vi "Main.vi"() -> ()   [LabVIEW 2013]
uses:
  ctrl/TYPE User Event.ctl
  <vilib>/Utility/miscctls.llb/LVComboBoxStrsAndValuesArrayTypeDef.ctl
  <vilib>/Utility/error.llb/whitespace.ctl
  <vilib>/Utility/miscctls.llb/LVTextColorsTypeDef.ctl
  <vilib>/Utility/miscctls.llb/LVRowAndColumnUnsignedTypeDef.ctl
  <vilib>/Utility/file.llb/Read From Spreadsheet File (string).vi
panel:
  in  "Tab Control":enum32{"股票价格历史数据图", "股票实时数据图"}(tab)
  out "Date":string
  out "Name":string
  in  "Right":bool
  in  "Left":bool
  out "股票价格历史数据图":cluster{i32[], dbl[]}[](graph)
  in  "停止":bool
  out "时间":string
  out "当天股价实时曲线":dbl[][](graph)
  out "卖1竞价":dbl format="%.2g"
  out "买1竞价":dbl format="%.2g"
  out "卖1至5总量":dbl
  out "买1至5总量":dbl
  out "今日最低":dbl format="%.2f"
  out "今日最高":dbl format="%.2f"
  out "昨日收盘":dbl format="%.2f"
  out "今日开盘":dbl format="%.2f"
  out "当前股价":dbl format="%.2f"
  out "BuySellBar":cluster{dbl[], dbl[]}[](graph)
  out "当前%":dbl format="%.2g%%"
  in  "Up":bool
  in  "Down":bool
  in  "读取类型":enum32{"股票列表", "数据记录"}(tab)
  in  "股票代码查询":string(combo)
  in  "股票列表":i32(listbox)
  in  "股票文件列表":i32(listbox)
  out "股票数据路径":path
  in  "起始日期":timestamp=timestamp(3408258341.818551 s since 1904-01-01) format="%<%Y/%m/%d>T"
  in  "终止日期":timestamp format="%<%Y/%m/%d>T"
  # "起始日期"
  # "截止日期"
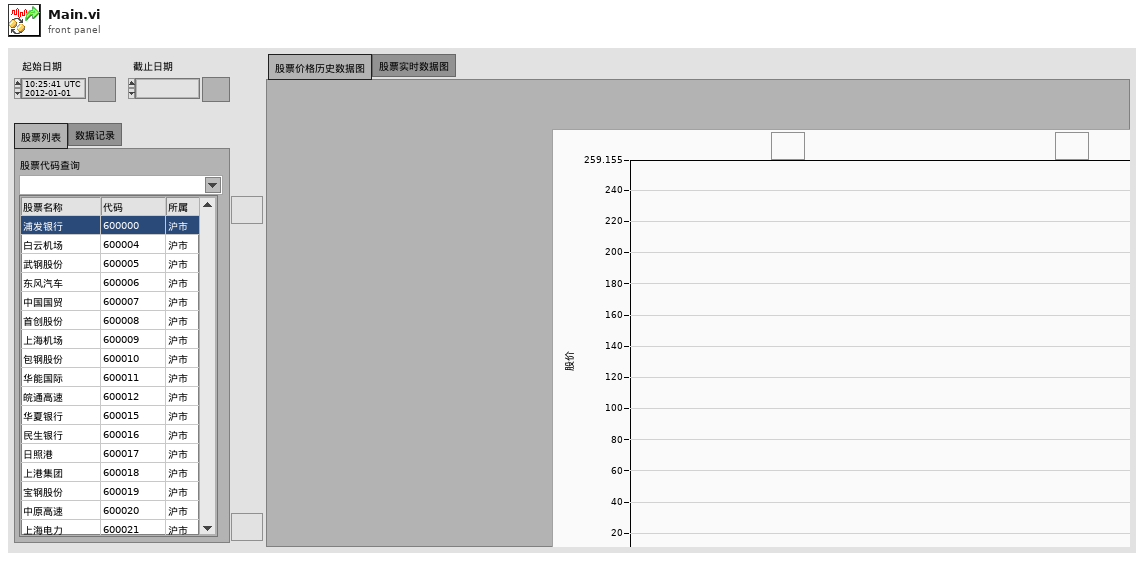
[diagram p1: front panel]
types:
  T1 = typedef "TYPE User Event.ctl" = cluster{"CMD":string, "Data":variant}
  T2 = cluster{"今日开盘":refnum<vi>, "昨日收盘":refnum<vi>, "当前股价":refnum<vi>, "今日最高":refnum<vi>, "今日最低":refnum<vi>, "买1竞价":refnum<vi>, "卖1竞价":refnum<vi>, "买1至5总量":refnum<vi>, "卖1至5总量":refnum<vi>, "当前%":refnum<vi>}
  T3 = typedef "LVComboBoxStrsAndValuesArrayTypeDef.ctl" = cluster{"String":string, "Value":string}[]
  T4 = typedef "LVTextColorsTypeDef.ctl" = cluster{"Text Color":u32, "Background Color":u32}
  T5 = typedef "LVRowAndColumnUnsignedTypeDef.ctl" = cluster{"Row":u32, "Column":u32}
  T6 = typedef "whitespace.ctl" = u16
  T7 = typedef "TYPE Price.ctl" = cluster{"Price":cluster{"Open":dbl, "Close":dbl, "Current":dbl, "High":dbl, "Low":dbl, "Buy1":dbl, "Sell1":dbl, "Total":dbl, "Account":dbl}, "Percent":dbl, "TotalBuy":dbl, "TotalSell":dbl, "TimeStamp":string}
  T8 = typedef "LVPoint32TypeDef.ctl" = cluster{"Horizontal":i32, "Vertical":i32}
  T9 = typedef "LVCursorListTypeDef.ctl" = cluster{"Name":string, "Color":u32, "Style":u8, "Point Style":u8, "Name Visible":bool, "Allow Drag":bool, "Cursor Mode":u32, "Plot":i32, "Index":i32, "Position":cluster{"X":dbl, "Y":dbl}, "X Scale":u32, "Y Scale":u32, "Watch Plots":i32[], "Watch All Plots":bool, "Plot Area":i32, "Label Offset":cluster{"X":dbl, "Y":dbl}}[]
  T10 = cluster{"Name":string, "Color":u32, "Style":u8, "Point Style":u8, "Name Visible":bool, "Allow Drag":bool, "Cursor Mode":u32, "Plot":i32, "Index":i32, "Position":cluster{"X":dbl, "Y":dbl}, "X Scale":u32, "Y Scale":u32, "Watch Plots":i32[], "Watch All Plots":bool, "Plot Area":i32, "Label Offset":cluster{"X":dbl, "Y":dbl}}
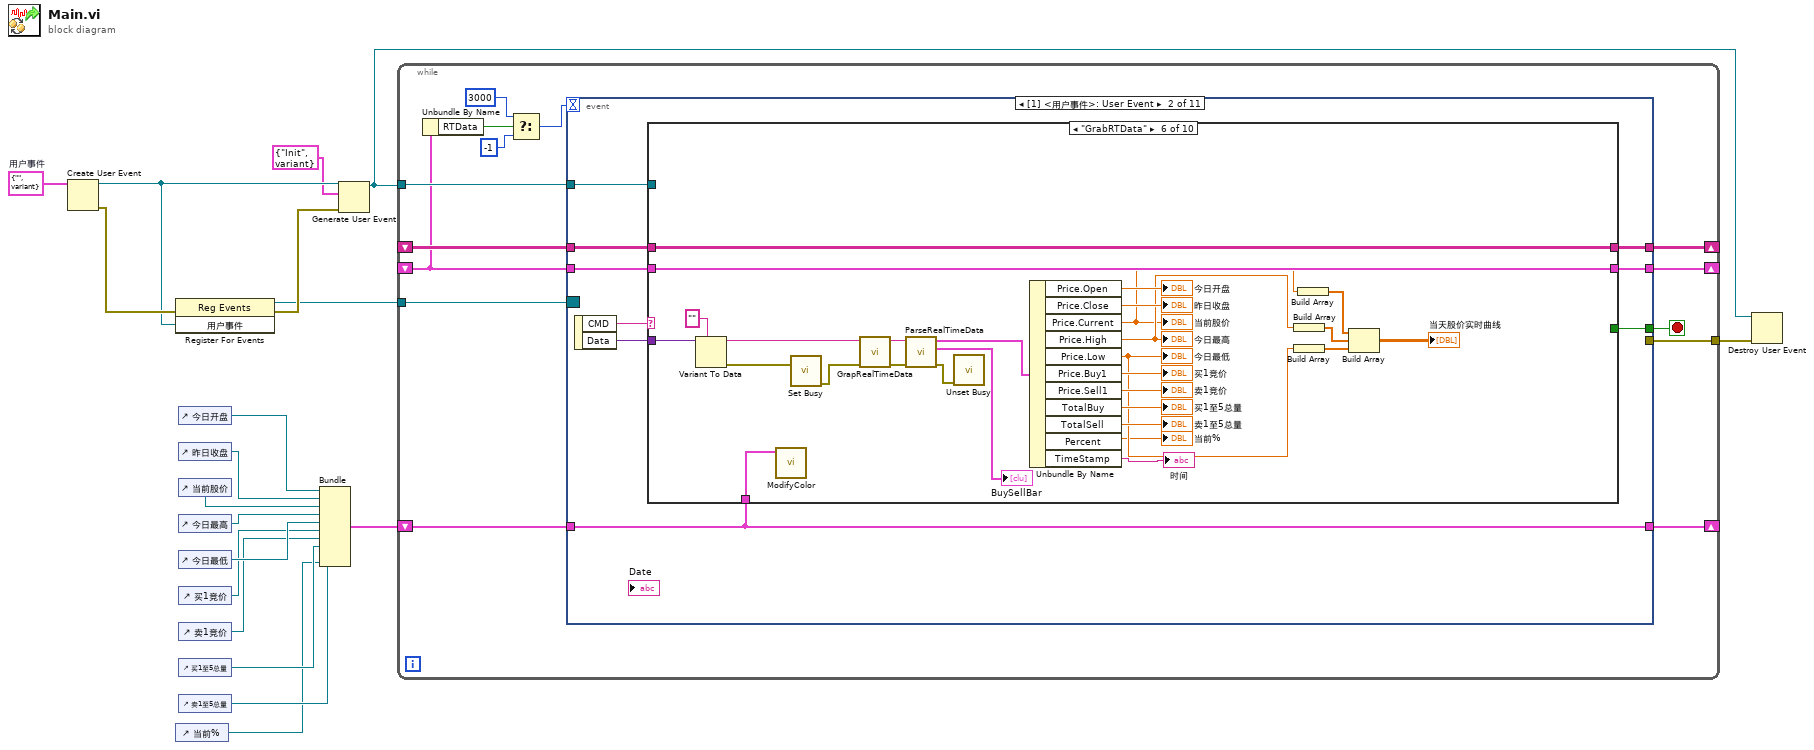
[diagram p0: block diagram]
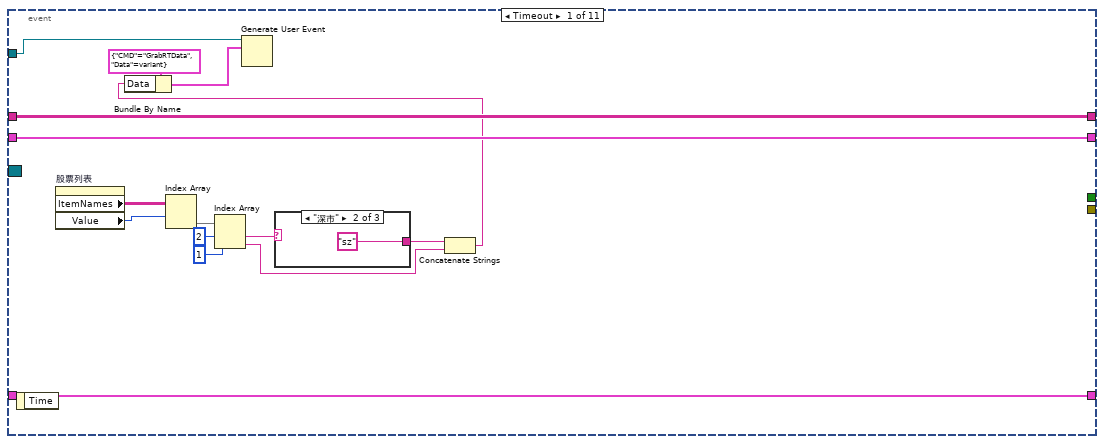
[diagram p2: hidden frame]
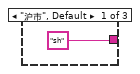
[diagram p3: hidden frame]
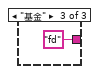
[diagram p4: hidden frame]
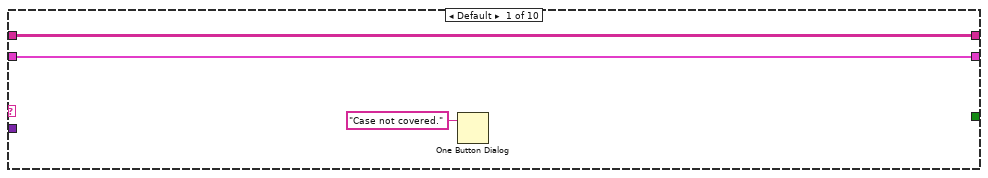
[diagram p5: hidden frame]
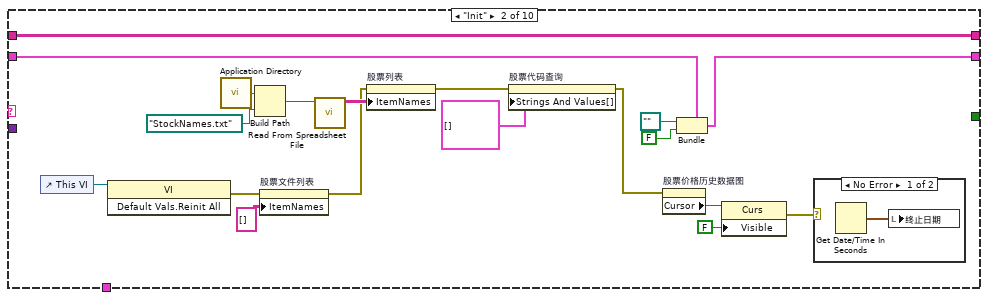
[diagram p6: hidden frame]
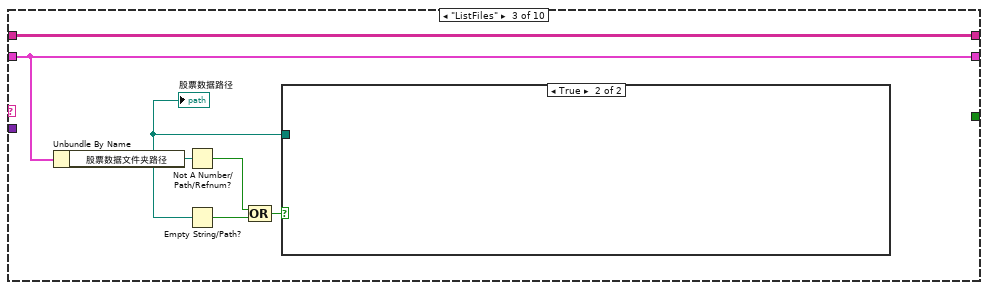
[diagram p8: hidden frame]
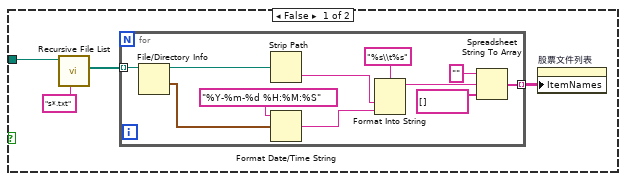
[diagram p9: hidden frame]
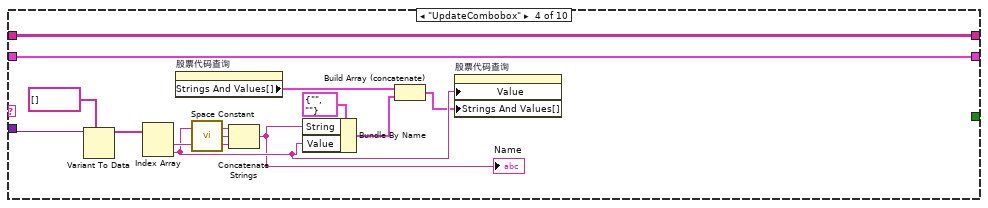
[diagram p10: hidden frame]
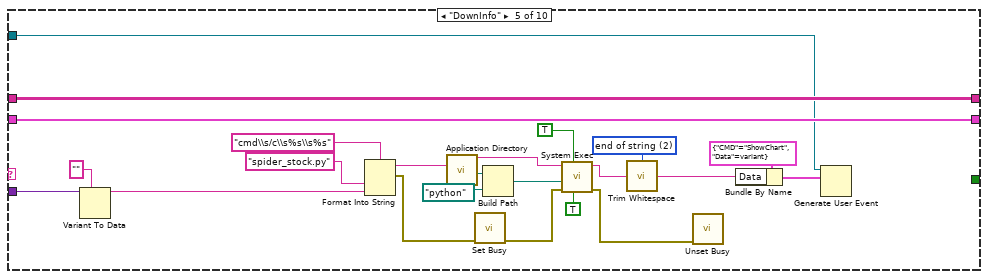
[diagram p11: hidden frame]
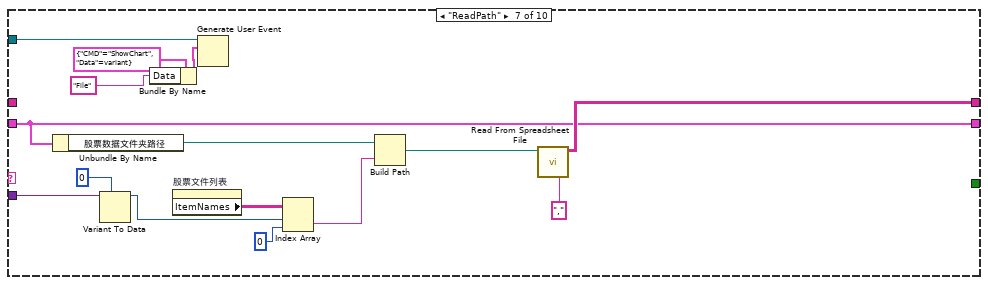
[diagram p12: hidden frame]
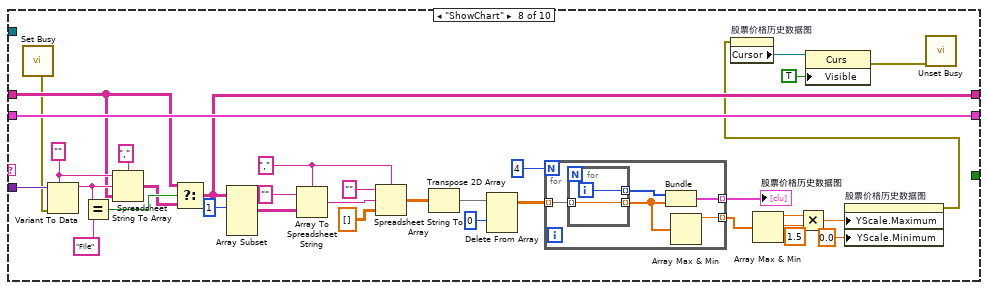
[diagram p13: hidden frame]
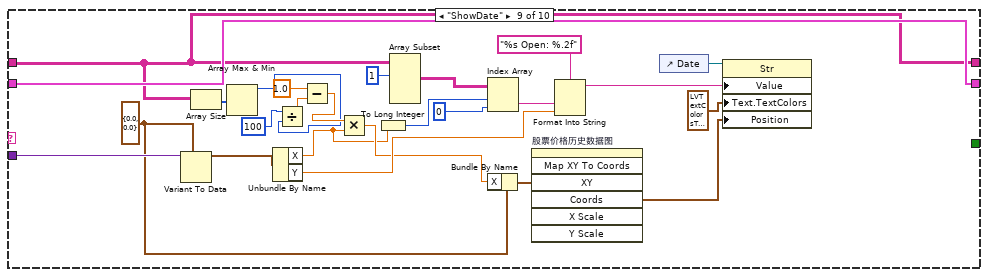
[diagram p14: hidden frame]
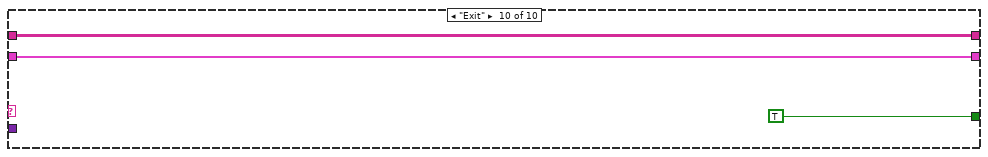
[diagram p15: hidden frame]
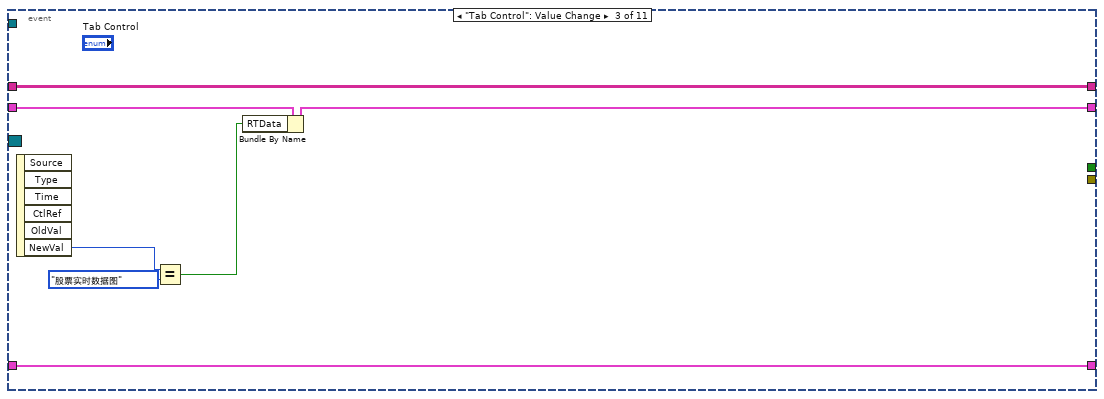
[diagram p16: hidden frame]
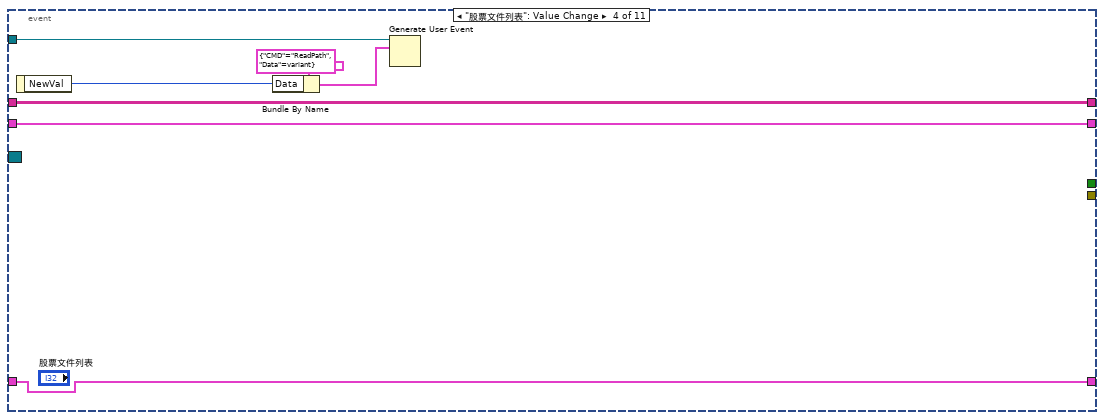
[diagram p17: hidden frame]
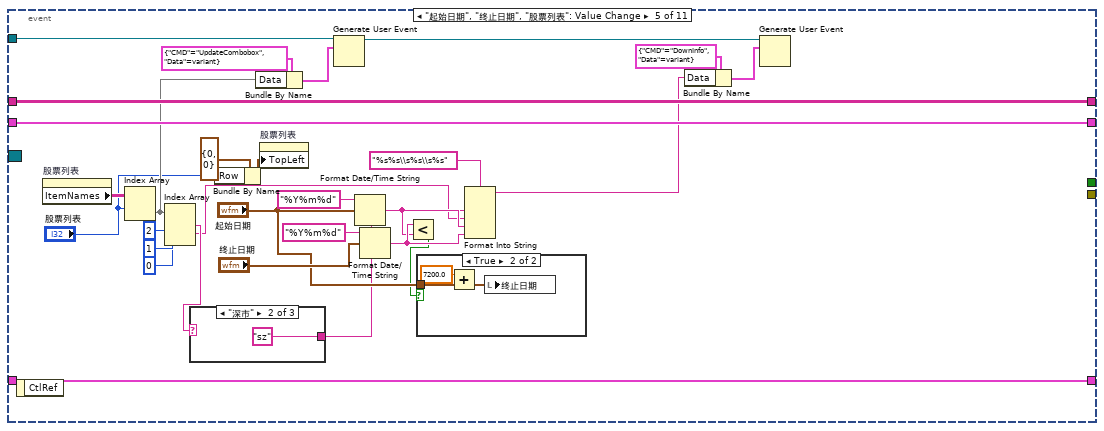
[diagram p18: hidden frame]
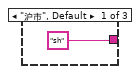
[diagram p19: hidden frame]
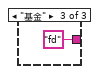
[diagram p20: hidden frame]
diagram:
  w15 = T1 {"CMD"="", "Data"=variant}  # 用户事件
  n1 = Create User Event(user event datatype=w15) -> (user event=w14:refnum<user-event>, error out=w18:errorcluster)  [unwired: 1 in]
  n2 = register-events(error in=w18, w14) -> (reference out=w17:refnum<event-registration>, error out=w19:errorcluster)  [unwired: 1 in]
  n3 = control-ref of="当前%"() -> (w1:refnum<vi>)
  n4 = control-ref of="今日开盘"() -> (w11:refnum<vi>)
  n5 = control-ref of="昨日收盘"() -> (w10:refnum<vi>)
  n6 = control-ref of="当前股价"() -> (w9:refnum<vi>)
  n7 = control-ref of="今日最高"() -> (w8:refnum<vi>)
  n8 = control-ref of="今日最低"() -> (w7:refnum<vi>)
  n9 = control-ref of="买1竞价"() -> (w6:refnum<vi>)
  n10 = control-ref of="卖1竞价"() -> (w5:refnum<vi>)
  n11 = control-ref of="买1至5总量"() -> (w4:refnum<vi>)
  n12 = control-ref of="卖1至5总量"() -> (w3:refnum<vi>)
  n13 = Bundle("今日开盘"=w11, "昨日收盘"=w10, "当前股价"=w9, "今日最高"=w8, "今日最低"=w7, "买1竞价"=w6, "卖1竞价"=w5, "买1至5总量"=w4, "卖1至5总量"=w3, "当前%"=w1) -> (w2:T2)  [unwired: 1 in]
  n14 = Generate User Event(user event=w14, event data cluster=T1 {"CMD"="Init", "Data"=variant} ("UsrEvent"), error in=w19) -> (user event out=w12:refnum<user-event>)  [unwired: 1 in, 1 out]
  n15 = while {
    shift-right: [w33] -> _
    shift-left: _ -> [w32]
    tunnel: w17 -> [w31]
    tunnel: w12 -> [w30]
    tunnel: [w29] -> w16
    shift-right: [w27] -> _
    shift-left: _ -> [w26]
    shift-right: [w21] -> _
    shift-left: w2 -> [w20]
    stop <- w28 stop-if-true
    n16 = Unbundle By Name(w26) -> ("RTData"=w24:bool)
    n17 = Select(t=3000, s=w24, f=-1) -> (s? t:f=w22:i32)
    n18 = event shown="[1] <用户事件>: User Event" {
      selector: w31 -> [_ _ _ _ _ _ _ _ _ _ _]
      dyn-events: _ -> [_ _ _ _ _ _ _ _ _ _ _]
      timeout: w22 -> [_ _ _ _ _ _ _ _ _ _ _]
      tunnel: [w48 w56 w257 w264 w293 w308 w324 w341 w358 w381 w390] -> w33
      tunnel: w32 -> [w48 w57 w257 w264 w293 w308 w324 w341 w358 w381 w390]
      tunnel: w30 -> [w44 w55 _ w262 w270 _ w313 w340 w354 _ w389]
      tunnel: [_ _ _ _ _ _ w312 _ _ _ _] -> w29
      tunnel: [_ w58 _ _ _ _ _ _ _ _ _] -> w28
      tunnel: w26 -> [w47 w54 w256 w259 w292 w307 w320 w336 w357 w380 w387]
      tunnel: [w47 w53 w253 w259 w292 w307 w321 w336 w357 w380 w387] -> w27
      tunnel: [w34 w52 w251 w258 w265 w300 w310 w334 w342 w375 w386] -> w21
      tunnel: w20 -> [w34 w52 w251 w258 w265 w300 w310 w334 w342 w375 w386]
      event Timeout {
        n19 = event-data() -> ()  [unwired: 1 in, 1 out]
        n20 = property on="股票列表" class="MCListbox (strict)"() -> ("ItemNames"=w43:string[][], "Value"=w42:i32)  [unwired: 2 in, 2 out]
        n21 = Index Array(array=w43, index (row)=w42) -> (element=w41:string[])  [unwired: 1 in]
        n22 = Index Array(array=w41, index #1=2 ("index"), index #2=1 ("index")) -> (element #1=w39:string, element #2=w36:string)
        n23 = case shown="\"深市\"" w39 {
          tunnel: ["sh" ("代码") "sz" ("代码") "fd" ("代码")] -> w37
          frame "沪市", Default {
          }
          frame "深市" {
          }
          frame "基金" {
          }
        }
        n24 = Concatenate Strings(w37, w36) -> (w35:string)
        n25 = Bundle By Name(cluster=T1 {"CMD"="GrabRTData", "Data"=variant} ("UsrEvent"), "Data"=w35) -> (w45:T1)
        n26 = Generate User Event(user event=w44, event data cluster=w45) -> ()  [unwired: 2 in, 2 out]
      }
      event User Event {
        n27 = event-data() -> ("CMD"=w60:string, "Data"=w59:variant)  [unwired: 1 in]
        n28 = case shown="\"GrabRTData\"" w60 {
          tunnel: w57 -> [w63 w82 w89 w117 w139 w167 _ w194 w231 w249]
          tunnel: w59 -> [_ _ _ w115 w133 w164 w180 w200 w246 _]
          tunnel: [_ _ _ _ _ _ _ _ _ TRUE] -> w58
          tunnel: [w63 w82 w89 w117 w139 w167 w182 w192 w231 w249] -> w56
          tunnel: w55 -> [_ _ _ _ w129 _ w181 _ _ _]
          tunnel: w54 -> [w62 w78 w88 w116 w138 w166 w174 w203 w240 w248]
          tunnel: [w62 w77 w88 w116 w138 w166 w174 w203 w240 w248] -> w53
          tunnel: w52 -> [_ _ _ _ _ w142 _ _ _ _]
          frame Default {
            n29 = One Button Dialog(message="Case not covered.") -> ()  [unwired: 1 in, 1 out]
          }
          frame "Init" {
            n30 = control-ref of="This VI"() -> (w80:refnum<vi>)
            n31 = invoke class="VI" method="Default Vals.Reinit All"(reference=w80) -> (error out=w79:errorcluster)  [unwired: 2 in, 2 out]
            n32 = call <vilib>:"Application Directory.vi"() -> ("Application Directory"=w71:path)
            n33 = Build Path(base path=w71, name or relative path=path "StockNames.txt" ("file path (dialog if empty)")) -> (appended path=w69:path)
            n34 = property on="股票文件列表" class="MCListbox (strict)"(error in=w79, "ItemNames"=string[][] [] ("Item Names")) -> (error out=w66:errorcluster)  [unwired: 1 in, 1 out]
            n35 = call-poly <vilib>:"Read From Spreadsheet File.vi"("file path (dialog if empty)"=w69) -> ("all rows"=w72:string[][])  [unwired: 6 in, 4 out]
            n36 = property on="股票列表" class="MCListbox (strict)"(error in=w66, "ItemNames"=w72) -> (error out=w67:errorcluster)  [unwired: 1 in, 1 out]
            n37 = property on="股票代码查询" class="CmbBox"(error in=w67, "Strings And Values[]"=T3 [] ("Strings And Values []")) -> (error out=w65:errorcluster)  [unwired: 1 in, 1 out]
            n38 = property on="股票价格历史数据图" class="XYGraph (strict)"(error in=w65) -> ("Cursor"=w75:refnum<vi>)  [unwired: 1 in, 2 out]
            n39 = Bundle(cluster=w78, "股票数据文件夹路径"=path "", "RTData"=FALSE) -> (w77:cluster{"股票数据文件夹路径":path, "RTData":bool})
            n40 = property class="Curs"(reference=w75, "Visible"=FALSE) -> (error out=w73:errorcluster)  [unwired: 1 in, 1 out]
            n41 = case shown="No Error" w73 {
              frame No Error {
                n42 = Get Date/Time In Seconds() -> (seconds since 1Jan1904=w83:timestamp)
                n43 = local write "终止日期"(w83) -> ()
              }
              frame Error {
              }
            }
          }
          frame "ListFiles" {
            n44 = Unbundle By Name(w88) -> ("股票数据文件夹路径"=w84:path)
            "股票数据路径" <- w84
            n45 = Not A Number/Path/Refnum?(number/path/refnum=w84) -> (NaN/Path/Refnum?=w86:bool)
            n46 = Empty String/Path?(string/path=w84) -> (empty?=w87:bool)
            n47 = Compound Arithmetic op=OR(w86, w87) -> (w85:bool)
            n48 = case shown="True" w85 {
              tunnel: w84 -> [w90 _]
              frame False {
                n49 = call <vilib>:"Recursive File List.vi"("pattern"="s*.txt", "Folder Path"=w90) -> ("All Files in Dir"=w92:path[])  [unwired: 5 in, 4 out]
                n50 = for {
                  tunnel: w92 -> [w104] mode=indexing
                  tunnel: [w98] -> w91 mode=indexing
                  n51 = File/Directory Info(path=w104) -> (path out=w103:path, last mod=w102:timestamp)  [unwired: 1 in, 5 out]
                  n52 = Strip Path(path=w103) -> (name=w96:string)  [unwired: 1 out]
                  n53 = Format Date/Time String(time format string (%c)="%Y-%m-%d %H:%M:%S", seconds (now)=w102) -> (date/time string=w95:string)  [unwired: 1 in]
                  n54 = Format Into String(format string="%s\\t%s", w96, w95) -> (resulting string=w99:string)  [unwired: 2 in, 1 out]
                  n55 = Spreadsheet String To Array(format string="", spreadsheet string=w99, array type (2D Dbl)=string[] []) -> (array=w98:string[])  [unwired: 1 in]
                }
                n56 = property on="股票文件列表" class="MCListbox (strict)"("ItemNames"=w91) -> ()  [unwired: 2 in, 2 out]
              }
              frame True {
              }
            }
          }
          frame "UpdateCombobox" {
            n57 = Variant To Data(type=string[] [] ("subarray"), Variant=w115) -> (data=w113:string[])  [unwired: 1 in, 1 out]
            n58 = Index Array(array=w113) -> (element #1=w109:string, element #2=w107:string)  [unwired: 2 in]
            n59 = property on="股票代码查询" class="CmbBox"() -> ("Strings And Values[]"=w111:T3)  [unwired: 2 in, 2 out]
            n60 = call <vilib>:"Space Constant.vi"() -> ("String"=w108:string)
            n61 = Concatenate Strings(w107, w108, w109) -> (w105:string)
            "Name" <- w105
            n62 = Bundle By Name(cluster=cluster{"String":string, "Value":string} {"String"="", "Value"=""}, "String"=w105, "Value"=w107) -> (w110:cluster{"String":string, "Value":string})
            n63 = Build Array (concatenate)(w111, w110) -> (w106:T3)
            n64 = property on="股票代码查询" class="CmbBox"("Value"=w107, "Strings And Values[]"=w106) -> ()  [unwired: 2 in, 2 out]
          }
          frame "DownInfo" {
            w124 = T6 2 items=["both", "start of string", "end of string"] ("location (both)")
            n65 = Variant To Data(type="", Variant=w133) -> (data=w131:string)  [unwired: 1 in, 1 out]
            n66 = Format Into String(format string="cmd\\s/c\\s%s\\s%s", "spider_stock.py" ("input 1"), w131) -> (resulting string=w134:string, error out=w123:errorcluster)  [unwired: 2 in]
            n67 = call <vilib>:"Application Directory.vi"() -> ("Application Directory"=w120:path)
            n68 = call <vilib>:"Set Busy.vi"("error in (no error)"=w123) -> ("error out"=w122:errorcluster)  [unwired: 9 in, 1 out]
            n69 = Build Path(base path=w120, name or relative path=path "python" ("working directory")) -> (appended path=w118:path)
            n70 = call <vilib>:"System Exec.vi"("run minimized? (F)"=TRUE, "wait until completion? (T)"=TRUE, "error in (no error)"=w122, "working directory"=w118, "command line"=w134) -> ("error out"=w121:errorcluster, "standard output"=w126:string)  [unwired: 3 in, 2 out]
            n71 = call <vilib>:"Trim Whitespace.vi"("string"=w126, "location (both)"=w124) -> ("trimmed string"=w125:string)
            n72 = call <vilib>:"Unset Busy.vi"("error in (no error)"=w121) -> ()  [unwired: 10 in, 1 out]
            n73 = Bundle By Name(cluster=T1 {"CMD"="ShowChart", "Data"=variant} ("UsrEvent"), "Data"=w125) -> (w128:T1)
            n74 = Generate User Event(user event=w129, event data cluster=w128) -> ()  [unwired: 2 in, 2 out]
          }
          frame "GrabRTData" {
            n75 = Variant To Data(type="", Variant=w164) -> (data=w163:string, error out=w146:errorcluster)  [unwired: 1 in]
            n76 = call "ModifyColor.vi"("ControlRefsIn"=w142) -> ()  [unwired: 10 in, 1 out]
            n77 = call <vilib>:"Set Busy.vi"("error in (no error)"=w146) -> ("error out"=w145:errorcluster)  [unwired: 9 in, 1 out]
            n78 = call "GrapRealTimeData.vi"("error in (no error)"=w145, "Code"=w163) -> ("error out"=w144:errorcluster, "Grab Data"=w162:string)  [unwired: 8 in]
            n79 = call "ParseRealTimeData.vi"("error in (no error)"=w144, "Raw Data"=w162) -> ("error out"=w143:errorcluster, "BuySellBar"=→"BuySellBar":cluster{dbl[], dbl[]}[], "Price"=w161:T7)  [unwired: 7 in]
            n80 = call <vilib>:"Unset Busy.vi"("error in (no error)"=w143) -> ()  [unwired: 10 in, 1 out]
            n81 = Unbundle By Name(w161) -> ("Price.Open"=→"今日开盘":dbl, "Price.Close"=→"昨日收盘":dbl, "Price.Current"=w149:dbl, "Price.High"=w154:dbl, "Price.Low"=w153:dbl, "Price.Buy1"=→"买1竞价":dbl, "Price.Sell1"=→"卖1竞价":dbl, "TotalBuy"=→"买1至5总量":dbl, "TotalSell"=→"卖1至5总量":dbl, "Percent"=→"当前%":dbl, "TimeStamp"=→"时间":string)
            "当前股价" <- w149
            "今日最低" <- w153
            "今日最高" <- w154
            n82 = Build Array(w154) -> (w151:dbl[])
            n83 = Build Array(w153) -> (w152:dbl[])
            n84 = Build Array(w149) -> (w148:dbl[])
            n85 = Build Array(w148, w151, w152) -> (→"当天股价实时曲线":dbl[][])
          }
          frame "ReadPath" {
            n86 = Unbundle By Name(w174) -> ("股票数据文件夹路径"=w173:path)
            n87 = Variant To Data(type=0, Variant=w180) -> (data=w177:i32)  [unwired: 1 in, 1 out]
            n88 = Bundle By Name(cluster=T1 {"CMD"="ShowChart", "Data"=variant} ("UsrEvent"), "Data"="File" ("CMD")) -> (w169:T1)
            n89 = property on="股票文件列表" class="MCListbox (strict)"() -> ("ItemNames"=w178:string[][])  [unwired: 2 in, 2 out]
            n90 = Generate User Event(user event=w181, event data cluster=w169) -> ()  [unwired: 2 in, 2 out]
            n91 = Index Array(array=w178, index (row)=w177, index (col)=0 ("disabled index (col)")) -> (element=w175:string)
            n92 = Build Path(base path=w173, name or relative path=w175) -> (appended path=w172:path)
            n93 = call-poly <vilib>:"Read From Spreadsheet File.vi"("delimiter (\\t)"="," ("delimiter (\\t)"), "file path (dialog if empty)"=w172) -> ("all rows"=w182:string[][])  [unwired: 5 in, 4 out]
          }
          frame "ShowChart" {
            w199 = "" ("Date")
            w206 = "," ("delimiter (Tab)")
            n94 = call <vilib>:"Set Busy.vi"() -> ("error out"=w184:errorcluster)  [unwired: 10 in, 1 out]
            n95 = Variant To Data(error in=w184, type=w199, Variant=w200) -> (data=w197:string)  [unwired: 1 out]
            n96 = Equal?(x=w197, y="File") -> (x = y?=w195:bool)
            n97 = Spreadsheet String To Array(delimiter (Tab)=",", format string=w199, spreadsheet string=w197, array type (2D Dbl)=w194) -> (array=w193:string[][])
            n98 = Select(t=w194, s=w195, f=w193) -> (s? t:f=w192:string[][])
            n99 = Array Subset(array=w192, index (row)=1 ("index")) -> (w215:string[][])  [unwired: 3 in]
            n100 = Array To Spreadsheet String(delimiter (Tab)=w206, array=w215, 3:"" ("format string")) -> (spreadsheet string=w205:string)
            n101 = Spreadsheet String To Array(delimiter (Tab)=w206, format string="", spreadsheet string=w205, array type (2D Dbl)=dbl[][] []) -> (array=w210:dbl[][])
            n102 = Transpose 2D Array(2D array=w210) -> (transposed array=w213:dbl[][])
            n103 = Delete From Array(array=w213, index (row)=0) -> (array with subset deleted=w190:dbl[][])  [unwired: 2 in, 1 out]
            n104 = for {
              N: 4 -> [_]
              tunnel: w190 -> [w220] mode=indexing
              tunnel: [w218] -> w211 mode=indexing
              tunnel: [w216] -> w189 mode=indexing
              n105 = for {
                tunnel: w220 -> [w221] mode=indexing
                tunnel: [w221] -> w217 mode=indexing
                tunnel: [w222] -> w219 mode=indexing
                i -> [w222]
              }
              n106 = Bundle(w219, w217) -> (w218:cluster{i32[], dbl[]})  [unwired: 1 in]
              n107 = Array Max & Min(array=w217) -> (max value=w216:dbl)  [unwired: 3 out]
            }
            "股票价格历史数据图" <- w211
            n108 = Array Max & Min(array=w189) -> (max value=w188:dbl)  [unwired: 3 out]
            n109 = Multiply(x=w188, y=1.5) -> (x*y=w187:dbl)
            n110 = property on="股票价格历史数据图" class="XYGraph (strict)"("YScale.Maximum"=w187, "YScale.Minimum"=0.0 ("Y Scale.Range:Minimum")) -> (error out=w185:errorcluster)  [unwired: 2 in, 1 out]
            n111 = property on="股票价格历史数据图" class="XYGraph (strict)"(error in=w185) -> ("Cursor"=w202:refnum<vi>)  [unwired: 1 in, 2 out]
            n112 = property class="Curs"(reference=w202, "Visible"=TRUE) -> (error out=w183:errorcluster)  [unwired: 1 in, 1 out]
            n113 = call <vilib>:"Unset Busy.vi"("error in (no error)"=w183) -> ()  [unwired: 10 in, 1 out]
          }
          frame "ShowDate" {
            w234 = cluster{"X":dbl, "Y":dbl} {"X"=0.0, "Y"=0.0} ("CursLoc")
            n114 = Variant To Data(type=w234, Variant=w246) -> (data=w233:cluster{"X":dbl, "Y":dbl})  [unwired: 1 in, 1 out]
            n115 = Array Size(array=w231) -> (size(s)=w230:i32[])
            n116 = Array Max & Min(array=w230) -> (max value=w223:i32)  [unwired: 3 out]
            n117 = Unbundle By Name(w233) -> ("X"=w225:dbl, "Y"=w232:dbl)
            n118 = Divide(x=100, y=w223) -> (x/y=w228:dbl)
            n119 = Subtract(x=1.0, y=w228) -> (x-y=w227:dbl)
            n120 = Multiply(x=w227, y=w225) -> (x*y=w226:dbl)
            n121 = To Long Integer(number=w225) -> (32bit integer=w242:i32)
            n122 = Array Subset(array=w231, index (row)=1 ("index")) -> (w243:string[][])  [unwired: 3 in]
            n123 = Index Array(array=w243, index (row)=w242, index (col)=0 ("disabled index (col)")) -> (element=w237:string)
            n124 = Bundle By Name(cluster=w234, "X"=w226) -> (w235:cluster{"X":dbl, "Y":dbl})
            n125 = invoke on="股票价格历史数据图" class="XYGraph (strict)" method="Map XY To Coords"("XY"=w235) -> ("Coords"=w239:T8)  [unwired: 6 in, 6 out]
            n126 = Format Into String(format string="%s Open: %.2f", w237, w232) -> (resulting string=w238:string)  [unwired: 2 in, 1 out]
            n127 = control-ref of="Date"() -> (w247:refnum<vi>)
            n128 = property class="Str"(reference=w247, "Value"=w238, "Text.TextColors"=T4 {"Text Color"=16777222, "Background Color"=16777216} ("Text.Text Colors"), "Position"=w239) -> ()  [unwired: 1 in, 2 out]
          }
          frame "Exit" {
          }
        }
      }
      event "Tab Control": Value Change {
        n129 = event-data() -> ("NewVal"=w255:enum32{"股票价格历史数据图", "股票实时数据图"})  [unwired: 1 in, 5 out]
        n130 = Equal?(x=w255, y=enum32{"股票价格历史数据图", "股票实时数据图"}."股票实时数据图") -> (x = y?=w252:bool)
        n131 = Bundle By Name(cluster=w256, "RTData"=w252) -> (w253:cluster{"股票数据文件夹路径":path, "RTData":bool})
      }
      event "股票文件列表": Value Change {
        n132 = event-data() -> ("NewVal"=w260:i32)  [unwired: 1 in]
        n133 = Bundle By Name(cluster=T1 {"CMD"="ReadPath", "Data"=variant} ("UsrEvent"), "Data"=w260) -> (w261:T1)
        n134 = Generate User Event(user event=w262, event data cluster=w261) -> ()  [unwired: 2 in, 2 out]
      }
      event "起始日期", "终止日期", "股票列表": Value Change {
        n135 = event-data() -> ()  [unwired: 1 in, 1 out]
        n136 = property on="股票列表" class="MCListbox (strict)"() -> ("ItemNames"=w280:string[][])  [unwired: 2 in, 2 out]
        n137 = Index Array(array=w280, index (row)="股票列表") -> (element=w271:string[])  [unwired: 1 in]
        n138 = Index Array(array=w271, index #1=2 ("index"), index #2=1 ("index"), index #3=0 ("index")) -> (element #1=w277:string, element #2=w274:string)  [unwired: 1 out]
        n139 = case shown="\"深市\"" w277 {
          tunnel: ["sh" ("代码") "sz" ("代码") "fd" ("代码")] -> w276
          frame "沪市", Default {
          }
          frame "深市" {
          }
          frame "基金" {
          }
        }
        n140 = Bundle By Name(cluster=T5 {"Row"=0, "Column"=0} ("Top Left Visible Cell"), "Row"="股票列表") -> (w267:T5)
        n141 = Bundle By Name(cluster=T1 {"CMD"="UpdateCombobox", "Data"=variant} ("UsrEvent"), "Data"=w271) -> (w272:T1)
        n142 = property on="股票列表" class="MCListbox (strict)"("TopLeft"=w267) -> ()  [unwired: 2 in, 2 out]
        n143 = Generate User Event(user event=w270, event data cluster=w272) -> (user event out=w269:refnum<user-event>)  [unwired: 2 in, 1 out]
        n144 = Format Date/Time String(time format string (%c)="%Y%m%d", seconds (now)="起始日期") -> (date/time string=w281:string)  [unwired: 1 in]
        n145 = Format Date/Time String(time format string (%c)="%Y%m%d", seconds (now)="终止日期") -> (date/time string=w284:string)  [unwired: 1 in]
        n146 = Less?(x=w284, y=w281) -> (x < y?=w282:bool)
        n147 = case shown="True" w282 {
          tunnel: "起始日期" -> [_ w299]
          frame False {
          }
          frame True {
            n148 = Add(x=7200.0, y=w299) -> (x+y=w298:timestamp)
            n149 = local write "终止日期"(w298) -> ()
          }
        }
        n150 = Format Into String(format string="%s%s\\s%s\\s%s", w276, w274, w281, w284) -> (resulting string=w285:string)  [unwired: 2 in, 1 out]
        n151 = Bundle By Name(cluster=T1 {"CMD"="DownInfo", "Data"=variant} ("UsrEvent"), "Data"=w285) -> (w286:T1)
        n152 = Generate User Event(user event=w269, event data cluster=w286) -> ()  [unwired: 2 in, 2 out]
      }
      event "股票代码查询": Value Change {
        n153 = event-data() -> ()  [unwired: 1 in, 1 out]
        n154 = property on="股票列表" class="MCListbox (strict)"() -> ("ItemNames"=w302:string[][])  [unwired: 2 in, 2 out]
        n155 = Index Array(array=w302, index (col)=1 ("disabled index (col)")) -> (element=w303:string[])  [unwired: 1 in]
        n156 = Search 1D Array(1D array=w303, element="股票代码查询") -> (index of element=w301:i32)  [unwired: 1 in]
        n157 = Greater Or Equal To 0?(x=w301) -> (x >= 0?=w304:bool)
        n158 = case shown="True" w304 {
          tunnel: w301 -> [_ w309]
          frame False {
          }
          frame True {
            n159 = property on="股票列表" class="MCListbox (strict)"("Val(Sgnl)"=w309) -> ()  [unwired: 2 in, 2 out]
          }
        }
      }
      event "读取类型": Value Change {
        n160 = event-data() -> ("NewVal"=w323:enum32{"股票列表", "数据记录"})  [unwired: 1 in]
        n161 = Unbundle By Name(w320) -> ("股票数据文件夹路径"=w317:path)
        n162 = Not A Number/Path/Refnum?(number/path/refnum=w317) -> (NaN/Path/Refnum?=w318:bool)
        n163 = Empty String/Path?(string/path=w317) -> (empty?=w319:bool)
        n164 = Compound Arithmetic op=OR(w318, w319) -> (w316:bool)
        n165 = Equal?(x=enum32{"股票列表", "数据记录"}."数据记录", y=w323) -> (x = y?=w314:bool)
        n166 = Compound Arithmetic op=AND(w316, w314) -> (w315:bool)
        n167 = case shown="True" w315 {
          tunnel: w320 -> [w329 w332]
          tunnel: [w329 w331] -> w321
          tunnel: [_ w330] -> w311
          frame False {
          }
          frame True {
            n168 = call "File Dialog"() -> ("selected path"=w333:path, "error out"=w330:errorcluster)  [unwired: 12 in, 2 out]
            n169 = Bundle By Name(cluster=w332, "股票数据文件夹路径"=w333) -> (w331:cluster{"股票数据文件夹路径":path, "RTData":bool})
          }
        }
        n170 = case shown="True" w314 {
          tunnel: w313 -> [_ w328]
          tunnel: [_ w327] -> w312
          tunnel: w311 -> [_ w325]
          frame False {
          }
          frame True {
            n171 = Generate User Event(user event=w328, event data cluster=T1 {"CMD"="ListFiles", "Data"=variant} ("UsrEvent"), error in=w325) -> (error out=w327:errorcluster)  [unwired: 1 in, 1 out]
          }
        }
      }
      event "股票价格历史数据图": Cursor Move {
        n172 = event-data() -> ("CursLoc"=w335:cluster{"X":dbl, "Y":dbl})  [unwired: 1 in]
        n173 = Bundle By Name(cluster=T1 {"CMD"="", "Data"=variant} ("UsrEvent"), "CMD"="ShowDate", "Data"=w335) -> (w337:T1)
        n174 = Generate User Event(user event=w340, event data cluster=w337) -> ()  [unwired: 2 in, 2 out]
      }
      event "Left", "Right": Value Change {
        n175 = event-data() -> ("CtlRef"=w353:refnum<vi>)  [unwired: 1 in, 3 out]
        n176 = property class="Bool"(reference=w353) -> ("Label.Text"=w352:string)  [unwired: 1 in, 2 out]
        n177 = property on="股票价格历史数据图" class="XYGraph (strict)"() -> (error out=w351:errorcluster, "CrsrList"=w348:T9)  [unwired: 2 in, 1 out]
        n178 = for {
          tunnel: w352 -> [w365]
          tunnel: [w364] -> w347 mode=indexing
          tunnel: w348 -> [w361] mode=indexing
          shift-right: [w362] -> w350
          shift-left: w351 -> [w363]
          tunnel: [w360] -> w346
          tunnel: [w359] -> w343
          n179 = in-place {
            in-place-border: w365 -> [w370]
            in-place-border: w363 -> [w368]
            in-place-border: [w368] -> w362
            in-place-border: [w367] -> w360
            in-place-border: [w366] -> w359
            n180 = in-place-cluster #1(w361) -> ("Position.X"=w369:dbl, "Position.Y"=w366:dbl)
            n181 = case shown="\"Right\", Default" w370 {
              tunnel: w369 -> [w372 w374]
              tunnel: [w371 w373] -> w367
              frame "Right", Default {
                n182 = Increment(x=w372) -> (x+1=w371:dbl)
              }
              frame "Left" {
                n183 = Decrement(x=w374) -> (x-1=w373:dbl)
              }
            }
            n184 = in-place-cluster #1("Position.X"=w367, "Position.Y"=w366) -> (w364:T10)
          }
        }
        n185 = property on="股票价格历史数据图" class="XYGraph (strict)"(error in=w350, "CrsrList"=w347) -> (error out=w349:errorcluster)  [unwired: 1 in, 1 out]
        n186 = Bundle By Name(cluster=cluster{"X":dbl, "Y":dbl} {"X"=0.0, "Y"=0.0} ("CursLoc"), "X"=w346, "Y"=w343) -> (w344:cluster{"X":dbl, "Y":dbl})
        n187 = Bundle By Name(cluster=T1 {"CMD"="ShowDate", "Data"=variant} ("UsrEvent"), "Data"=w344) -> (w355:T1)
        n188 = Generate User Event(user event=w354, event data cluster=w355, error in=w349) -> ()  [unwired: 1 in, 2 out]
      }
      event "Up", "Down": Value Change {
        n189 = event-data() -> ("CtlRef"=w379:refnum<vi>)  [unwired: 1 in, 5 out]
        n190 = property class="Bool"(reference=w379) -> ("Label.Text"=w378:string)  [unwired: 1 in, 2 out]
        n191 = property on="股票列表" class="MCListbox (strict)"() -> ("Value"=w377:i32)  [unwired: 2 in, 2 out]
        n192 = case shown="\"Down\", Default" w378 {
          tunnel: w377 -> [w383 w385]
          tunnel: [w382 w384] -> w376
          frame "Down", Default {
            n193 = Increment(x=w383) -> (x+1=w382:i32)
          }
          frame "Up" {
            n194 = Decrement(x=w385) -> (x-1=w384:i32)
          }
        }
        n195 = property on="股票列表" class="MCListbox (strict)"("Val(Sgnl)"=w376) -> ()  [unwired: 2 in, 2 out]
      }
      event "停止": Value Change {
        n196 = event-data() -> ()  [unwired: 1 in, 1 out]
        n197 = Generate User Event(user event=w389, event data cluster=T1 {"CMD"="Exit", "Data"=variant} ("UsrEvent")) -> ()  [unwired: 2 in, 2 out]
      }
    }
  }
  n198 = Destroy User Event(user event=w12, error in=w16) -> ()  [unwired: 1 out]
